vi "Video2Image.vi"(5 "AVI Refnum":T1, 6 "Init Base Image":bool, 7 "AVI File Path":path, 8 "error in (no error)":errorcluster, 9 "Running Index":i32, 10 "Start Index":i32, 11 "Image In":T2(plugin-control)) -> (0 "error out":errorcluster, 3 "Image Out":T2(plugin-control))   [LabVIEW 2013]
uses:
  <vilib>/vision/Avi.llb/IMAQ AVI2 Refnum.ctl
  <vilib>/Analysis/baseanly.llb/Normalize Matrix.vi
  <vilib>/addons/Multicore Analysis and Sparse Matrix/Signal Operation/_sigop/2D Cross Correlation (DBL).vi
  <vilib>/vision/NI_Vision_Development_Module.lvlib
  <vilib>/addons/Multicore Analysis and Sparse Matrix/Signal Operation/NI_MASM_SigOperation.lvlib
  <vilib>/Analysis/NI_AALBase.lvlib
panel:
  out "Result":dbl[][](graph)
  out "max index(es)":i32[](array[numeric])
  out "Changing image":dbl[][](graph)
  out "Ref":dbl[][](graph)
  out "x-1":i32[](array[numeric])
  out "Image":T2(plugin-control)
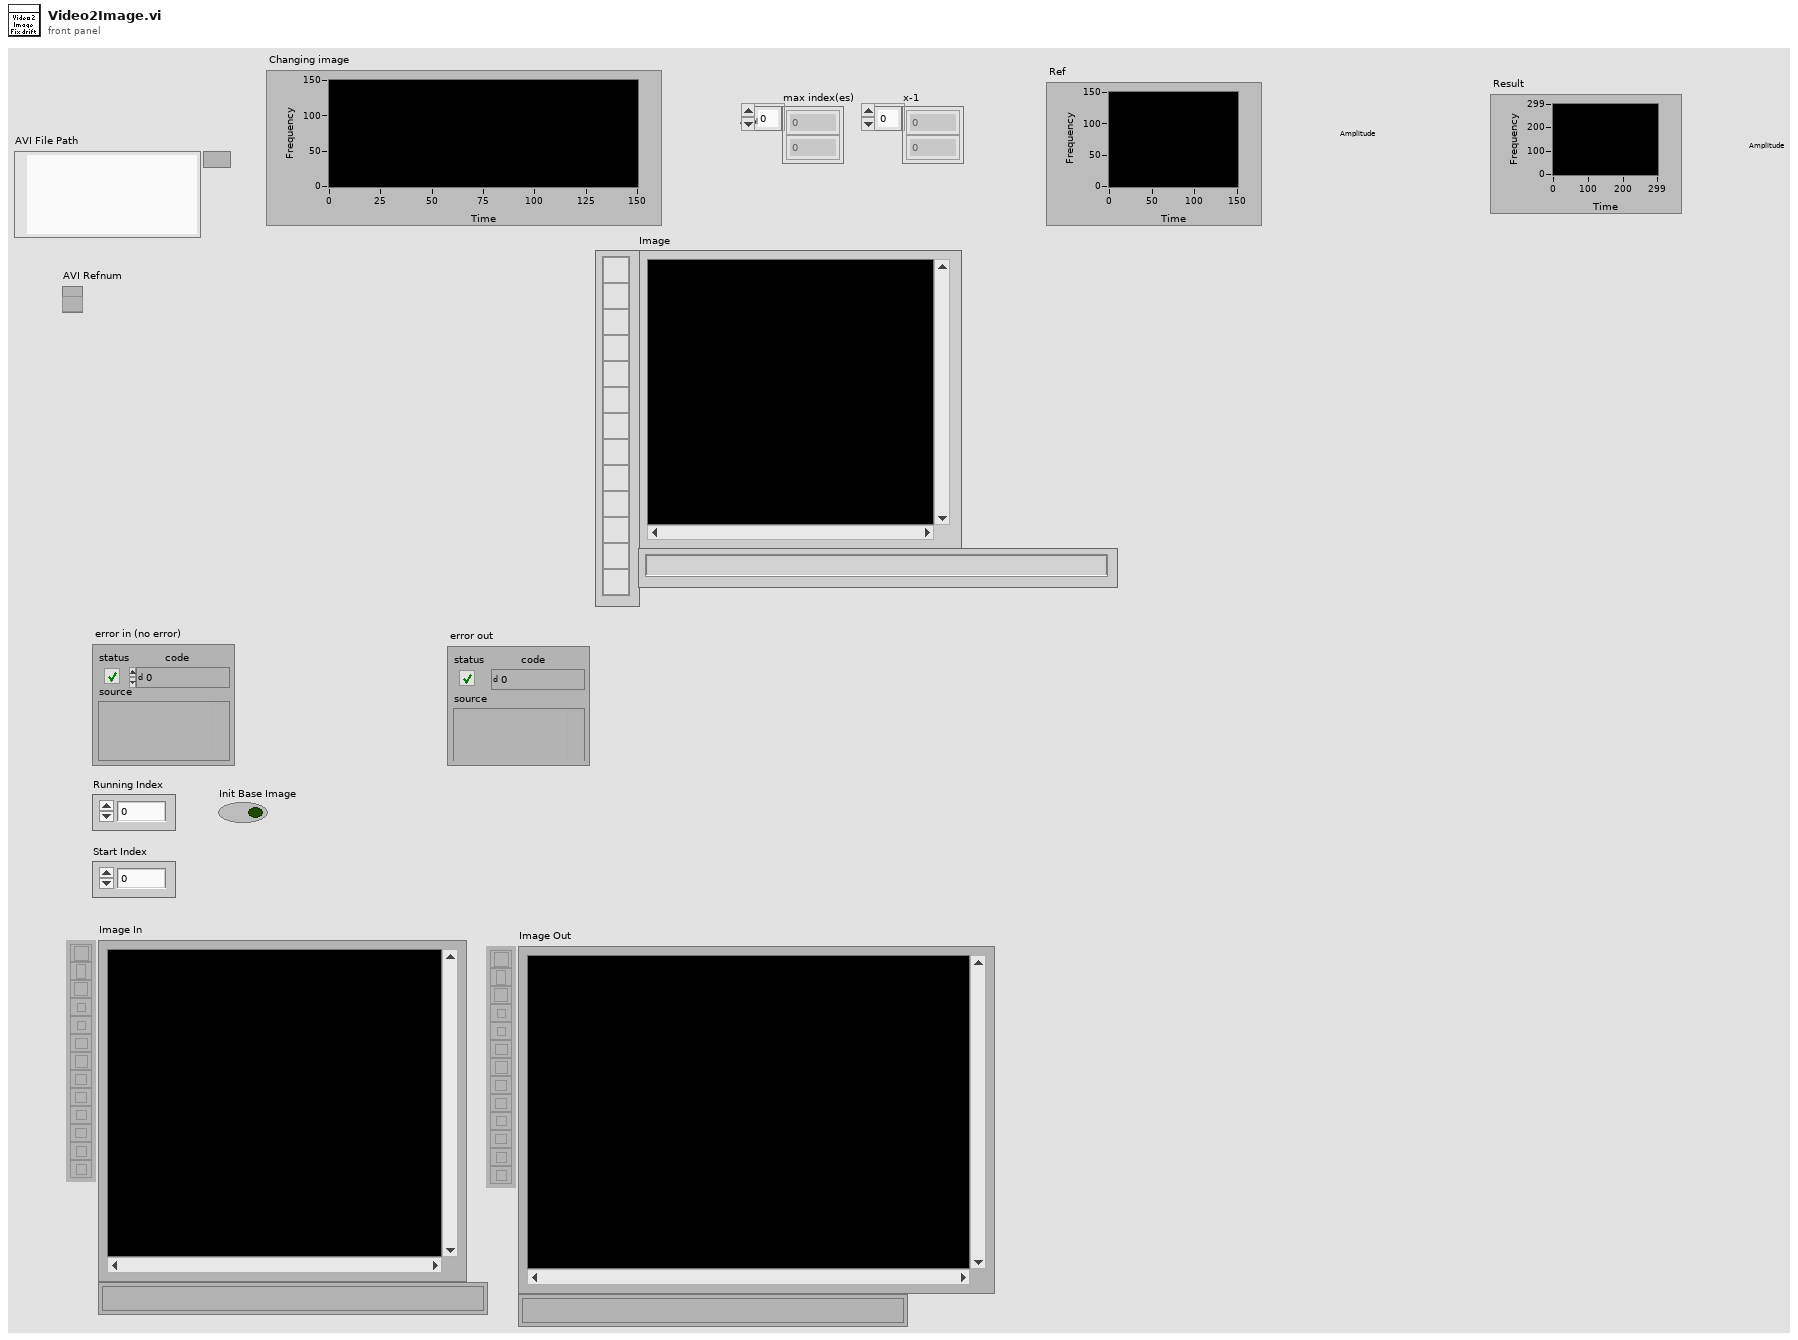
[diagram p1: front panel]
types:
  T1 = typedef "IMAQ AVI2 Refnum.ctl" = refnum<k20>
  T2 = typedef "IMAQ Image.ctl" = refnum<image>
  T3 = typedef "NI_Matrix.lvlib/RealMatrix.ctl" = dbl[][]
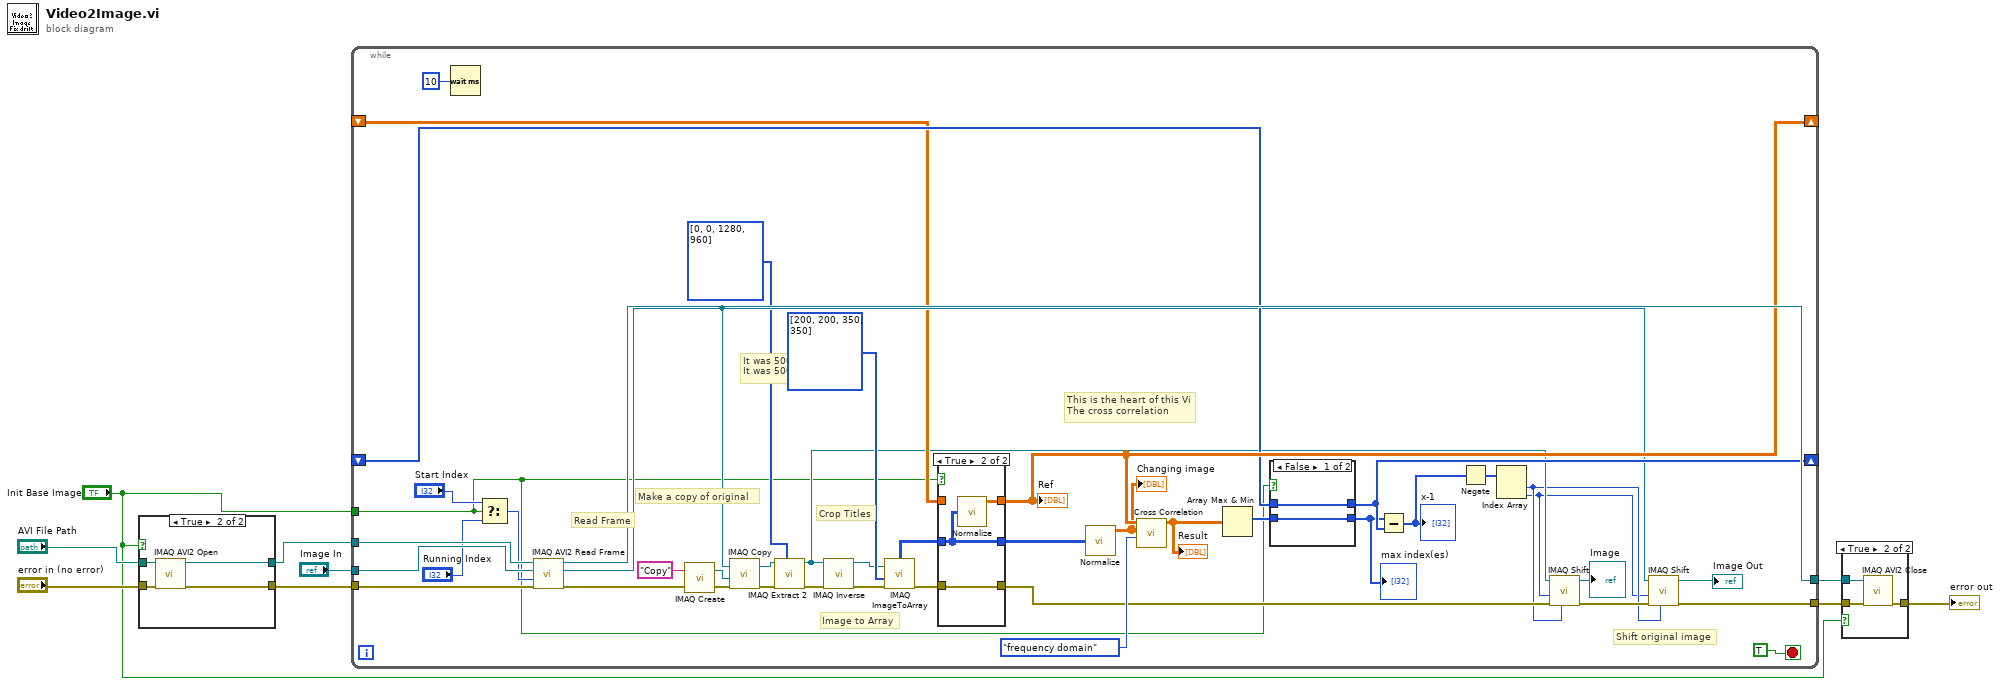
[diagram p0: block diagram]
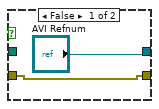
[diagram p3: hidden frame]
diagram:
  n1 = case shown="True" "Init Base Image" {
    tunnel: "AVI File Path" -> [_ w15]
    tunnel: ["AVI Refnum" w14] -> w5
    tunnel: [w10 w13] -> w4
    tunnel: "error in (no error)" -> [w10 w12]
    frame False {
    }
    frame True {
      n2 = call "IMAQ AVI2 Open"("error in (no error)"=w12, "AVI File Path"=w15) -> ("error out"=w13:errorcluster, "AVI Refnum"=w14:T1)  [unwired: 8 in]
    }
  }
  n3 = while {
    tunnel: w5 -> [w59]
    tunnel: w4 -> [w58]
    tunnel: "Image In" -> [w57]
    tunnel: [w56] -> w8
    tunnel: [w49] -> w7
    shift-right: [w54] -> _
    shift-left: _ -> [w47]
    shift-right: [w52] -> _
    shift-left: _ -> [w53]
    tunnel: "Init Base Image" -> [w16]
    stop <- TRUE stop-if-true
    # "It was 500\nIt was 500"
    # "Shift original image"
    # "Make a copy of original"
    # "This is the heart of this Vi\nThe cross correlation"
    # "Image to Array"
    # "Read Frame"
    # "Crop Titles"
    n4 = Wait (ms)(milliseconds to wait=u32 10) -> ()  [unwired: 1 out]
    n5 = Select(t="Start Index", s=w16, f="Running Index") -> (s? t:f=w44:i32)
    n6 = call "IMAQ AVI2 Read Frame"("error in (no error)"=w58, "Frame Number"=w44, "Image"=w57, "AVI Refnum"=w59) -> ("error out"=w50:errorcluster, "Image Out"=w48:T2, "AVI Refnum (duplicate)"=w56:T1)  [unwired: 5 in]
    n7 = call "IMAQ Create"("Image Name"="Copy", "error in (no error)"=w50) -> ("New Image"=w23:T2, "error out"=w24:errorcluster)  [unwired: 3 in]
    n8 = call "IMAQ Copy"("error in (no error)"=w24, "Image Dst"=w23, "Image Src"=w48) -> ("error out"=w21:errorcluster, "Image Dst Out"=w22:T2)  [unwired: 3 in]
    n9 = call "IMAQ Extract 2"("Optional Rectangle"=i32[] [0, 0, 1280, 960], "error in (no error)"=w21, "Image Src"=w22) -> ("error out"=w29:errorcluster, "Image Dst Out"=w26:T2)  [unwired: 7 in]
    n10 = call "IMAQ Inverse"("error in (no error)"=w29, "Image Src"=w26) -> ("error out"=w28:errorcluster, "Image Dst Out"=w27:T2)  [unwired: 8 in]
    n11 = call "IMAQ ImageToArray"("error in (no error)"=w28, "Optional Rectangle"=i32[] [200, 200, 350, 350], "Image"=w27) -> ("error out"=w39:errorcluster, "Image Pixels (U8)"=w41:u8[][])  [unwired: 1 in, 3 out]
    n12 = case shown="True" w16 {
      tunnel: w41 -> [w65 w67]
      tunnel: [w64 w66] -> w54
      tunnel: [w65 w67] -> w36
      tunnel: w47 -> [w64 _]
      tunnel: w39 -> [w63 w68]
      tunnel: [w63 w68] -> w20
      frame False {
      }
      frame True {
        n13 = call-poly <vilib>:"Normalize.vi"("Matrix"=w67) -> ("Normalized Matrix"=w66:T3)  [unwired: 1 in, 3 out]
      }
    }
    "Ref" <- w54
    n14 = call-poly <vilib>:"Normalize.vi"("Matrix"=w36) -> ("Normalized Matrix"=w35:T3)  [unwired: 1 in, 3 out]
    "Changing image" <- w35
    n15 = call-poly <vilib>:"Cross Correlation.vi"("algorithm"=enum32{"direct", "frequency domain"}."frequency domain", "Y"=w35, "X"=w54) -> ("Rxy"=w37:dbl[][])  [unwired: 7 in, 1 out]
    "Result" <- w37
    n16 = Array Max & Min(array=w37) -> (max index (indices)=w34:i32[])  [unwired: 3 out]
    n17 = case shown="False" w16 {
      tunnel: w34 -> [w60 w62]
      tunnel: [w61 w62] -> w52
      tunnel: w53 -> [w61 _]
      tunnel: [w60 w62] -> w33
      frame False {
      }
      frame True {
      }
    }
    "max index(es)" <- w33
    n18 = Subtract(x=w33, y=w52) -> (x-y=w31:i32[])
    "x-1" <- w31
    n19 = Negate(x=w31) -> (-x=w30:i32[])
    n20 = Index Array(array=w30) -> (element #1=w18:i32, element #2=w17:i32)  [unwired: 2 in]
    n21 = call "IMAQ Shift"("YOffset"=w18, "error in (no error)"=w20, "XOffset"=w17, "Image Src"=w26) -> ("error out"=w19:errorcluster, "Image Dst Out"=→"Image":T2)  [unwired: 6 in]
    n22 = call "IMAQ Shift"("YOffset"=w18, "error in (no error)"=w19, "XOffset"=w17, "Image Src"=w48) -> ("error out"=w49:errorcluster, "Image Dst Out"=→"Image Out":T2)  [unwired: 6 in]
  }
  n23 = case shown="True" "Init Base Image" {
    tunnel: w8 -> [_ w72]
    tunnel: w7 -> [w69 w71]
    tunnel: [w69 w70] -> w6
    frame False {
    }
    frame True {
      n24 = call "IMAQ AVI2 Close"("error in (no error)"=w71, "AVI Refnum"=w72) -> ("error out"=w70:errorcluster)  [unwired: 9 in]
    }
  }
  "error out" <- w6
